vi "Case_structure_for_temperature.vi"() -> ()   [LabVIEW 2019]
panel:
  in  "Input temp":dbl=-40.0
  out "Output":dbl
  in  "C or F":u16=1
  # "Put 1 for Celcius to Fahrenheit conversion\nand put 2 for Fahrenheit conversion.\nAny other value will be treated as default and\nwill give output 0."
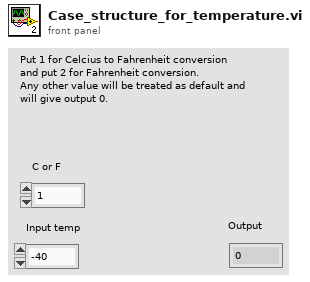
[diagram p1: front panel]
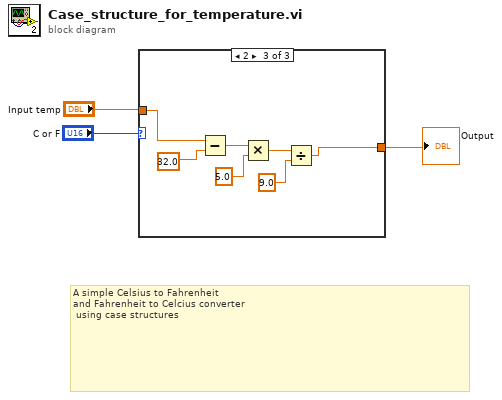
[diagram p0: block diagram]
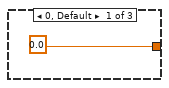
[diagram p2: hidden frame]
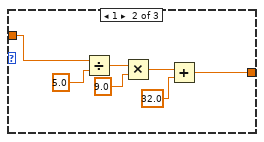
[diagram p3: hidden frame]
diagram:
  # "A simple Celsius to Fahrenheit\nand Fahrenheit to Celcius converter\n using case structures"
  n1 = case shown="2" "C or F" {
    tunnel: [0.0 w6 w13] -> w2
    tunnel: "Input temp" -> [_ w5 w12]
    frame 0, Default {
    }
    frame 1 {
      n2 = Divide(x=w5, y=5.0) -> (x/y=w10:dbl)
      n3 = Multiply(x=w10, y=9.0) -> (x*y=w8:dbl)
      n4 = Add(x=w8, y=32.0) -> (x+y=w6:dbl)
    }
    frame 2 {
      n5 = Subtract(x=w12, y=32.0) -> (x-y=w17:dbl)
      n6 = Multiply(x=w17, y=5.0) -> (x*y=w15:dbl)
      n7 = Divide(x=w15, y=9.0) -> (x/y=w13:dbl)
    }
  }
  "Output" <- w2
